vi "Main.Resize.vi"(10 "Sub Panel":refnum<vi>, 11 "VI in":refnum<vi>) -> ()   [LabVIEW 2019]
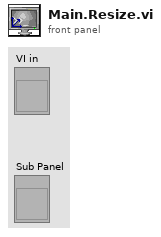
[diagram p1: front panel]
types:
  T1 = enum32{"Invalid", "Standard", "Closed", "Hidden", "Minimized", "Maximized"}
  T2 = typedef "LVAllMonitorsDisplayTypeDef.ctl" = cluster{"Bounds":cluster{"Left":i16, "Top":i16, "Right":i16, "Bottom":i16}, "Depth":i16}[]
  T3 = cluster{"Bounds":cluster{"Left":i16, "Top":i16, "Right":i16, "Bottom":i16}, "Depth":i16}
  T4 = cluster{"Left":i16, "Top":i16, "Right":i16, "Bottom":i16}
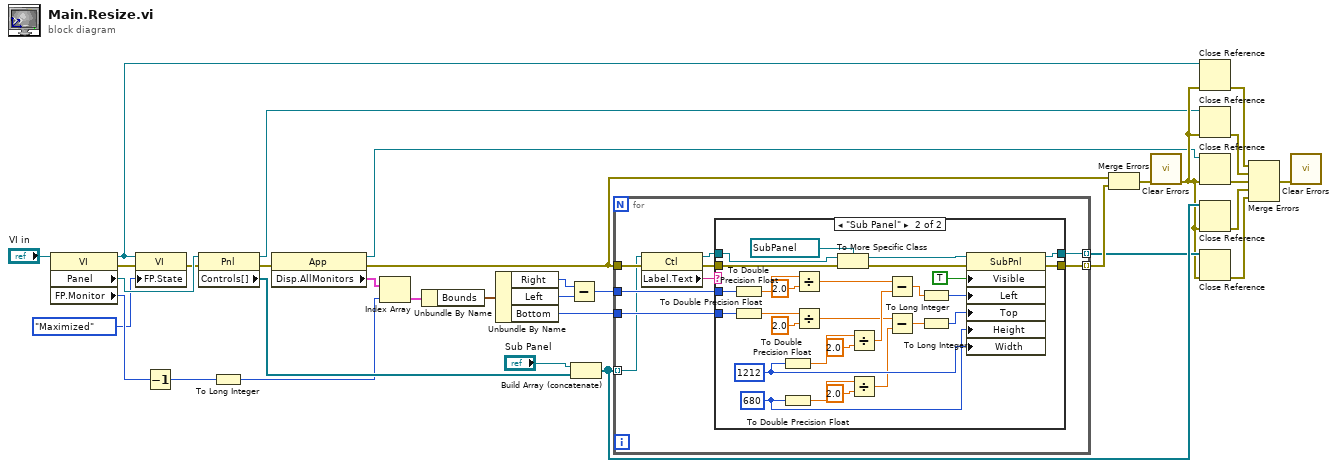
[diagram p0: block diagram]
diagram:
  n1 = property class="VI"(reference="VI in") -> (reference out=w1:refnum<vi>, error out=w3:errorcluster, "Panel"=w33:refnum<vi>, "FP.Monitor"=w31:u16)  [unwired: 1 in]
  n2 = property class="VI"(reference=w1, error in=w3, "FP.State"=T1."Maximized" ("Front Panel Window:State")) -> (error out=w2:errorcluster)  [unwired: 1 out]
  n3 = Decrement(x=w31) -> (x-1=w28:u16)
  n4 = property class="Pnl"(reference=w33, error in=w2) -> (reference out=w5:refnum<vi>, error out=w23:errorcluster, "Controls[]"=w20:refnum<vi>[])
  n5 = To Long Integer(number=w28) -> (32bit integer=w18:i32)
  n6 = property class="App"(error in=w23) -> (reference out=w6:refnum<vi>, error out=w11:errorcluster, "Disp.AllMonitors"=w32:T2)  [unwired: 1 in]
  n7 = Index Array(array=w32, index=w18) -> (element=w30:T3)
  n8 = Unbundle By Name(w30) -> ("Bounds"=w29:T4)
  n9 = Unbundle By Name(w29) -> ("Right"=w27:i16, "Left"=w26:i16, "Bottom"=w24:i16)
  n10 = Subtract(x=w27, y=w26) -> (x-y=w25:i16)
  n11 = Build Array (concatenate)("Sub Panel", w20) -> (w17:refnum<vi>[])
  n12 = for {
    tunnel: w25 -> [w42]
    tunnel: w24 -> [w41]
    tunnel: w17 -> [w35] mode=indexing
    tunnel: [w34] -> w15 mode=indexing
    tunnel: w11 -> [w36]
    tunnel: [w40] -> w22 mode=indexing
    n13 = property class="Ctl"(reference=w35, error in=w36) -> (reference out=w38:refnum<vi>, error out=w37:errorcluster, "Label.Text"=w39:string)
    n14 = case shown="\"Sub Panel\"" w39 {
      tunnel: w37 -> [w44 w69]
      tunnel: [w44 w66] -> w40
      tunnel: w38 -> [w43 w70]
      tunnel: w42 -> [_ w59]
      tunnel: w41 -> [_ w57]
      tunnel: [w43 w51] -> w34
      frame Default {
      }
      frame "Sub Panel" {
        w62 = u32 1212 ("Container Bounds:Width")
        w52 = u32 680 ("Container Bounds:Height")
        n15 = To Double Precision Float(number=w59) -> (double precision float=w48:dbl)
        n16 = To Double Precision Float(number=w57) -> (double precision float=w46:dbl)
        n17 = To Double Precision Float(number=w62) -> (double precision float=w47:dbl)
        n18 = To Double Precision Float(number=w52) -> (double precision float=w45:dbl)
        n19 = Divide(x=w48, y=2.0) -> (x/y=w64:dbl)
        n20 = Divide(x=w46, y=2.0) -> (x/y=w56:dbl)
        n21 = To More Specific Class(target class=refnum<vi> refnum ("reference"), reference=w70, error in=w69) -> (specific class reference=w67:refnum<vi>, error out=w68:errorcluster)
        n22 = Divide(x=w47, y=2.0) -> (x/y=w61:dbl)
        n23 = Divide(x=w45, y=2.0) -> (x/y=w54:dbl)
        n24 = Subtract(x=w64, y=w61) -> (x-y=w60:dbl)
        n25 = Subtract(x=w56, y=w54) -> (x-y=w53:dbl)
        n26 = To Long Integer(number=w60) -> (32bit integer=w49:i32)
        n27 = To Long Integer(number=w53) -> (32bit integer=w50:i32)
        n28 = property class="SubPnl"(reference=w67, error in=w68, "Visible"=TRUE, "Left"=w49, "Top"=w50, "Height"=w52, "Width"=w62) -> (reference out=w51:refnum<vi>, error out=w66:errorcluster)
      }
    }
  }
  n29 = Merge Errors(w11, w22) -> (w12:errorcluster)
  n30 = call <vilib>:"Clear Errors.vi"("error in (no error)"=w12) -> ("error out"=w10:errorcluster)  [unwired: 5 in, 1 out]
  n31 = Close Reference(reference=w1, error in (no error)=w10) -> (error out=w7:errorcluster)
  n32 = Close Reference(reference=w5, error in (no error)=w10) -> (error out=w8:errorcluster)
  n33 = Close Reference(reference=w6, error in (no error)=w10) -> (error out=w9:errorcluster)
  n34 = Close Reference(reference=w17, error in (no error)=w10) -> (error out=w16:errorcluster)
  n35 = Close Reference(reference=w15, error in (no error)=w10) -> (error out=w13:errorcluster)
  n36 = Merge Errors(w7, w8, w9, w16, w13) -> (w14:errorcluster)
  n37 = call <vilib>:"Clear Errors.vi"("error in (no error)"=w14) -> ()  [unwired: 5 in, 2 out]
